vi "Update VS channels - incoming - (object info).vi"(9 "reflectAttributeValues in":T1, 10 "hla map helpers in":T7, 11 "values in":dbl[](array[numeric])) -> (1 "reflectAttributeValues out":T1, 2 "hla map helpers out":T7, 3 "values out":dbl[](array[numeric]))   [LabVIEW 2019, in "HLA Custom Device Engine.lvlib"]
uses:
  HLA Custom Device Engine.lvlib
  _typedefs/RThlaMapHelpers.ctl
  _typedefs/map_in_interaction.ctl
  _typedefs/map_interaction_value.ctl
  _typedefs/map_attr_param_data.ctl
  _typedefs/map_object.ctl
  _typedefs/map_object_key.ctl
  _typedefs/map_object_value.ctl
  _typedefs/map_object_instance.ctl
  _typedefs/map_object_instance_value.ctl
  _typedefs/map_object_vs_instance.ctl
  _typedefs/map_out_vs_ch_instanceId.ctl
  _typedefs/map_out_vs_ch_objects.ctl
  _typedefs/map_out_vs_ch_objects_value.ctl
  _typedefs/map_out_vs_ch_interactIonClass.ctl
  _typedefs/reflectAttributeValues_type.ctl
  _typedefs/object_info_received_type.ctl
  <vilib>/addons/hla/TransportationType.ctl
  <vilib>/addons/hla/OrderType.ctl
  Shared/vs_obj_id_state.ctl
  _typedefs/dataElement_type.ctl
  _Debug/VsDebugLibrary.lvlib
  <vilib>/addons/hla/openrti_rti1516eLv.lvlib
  Shared/HLA Custom Device Shared.lvlib
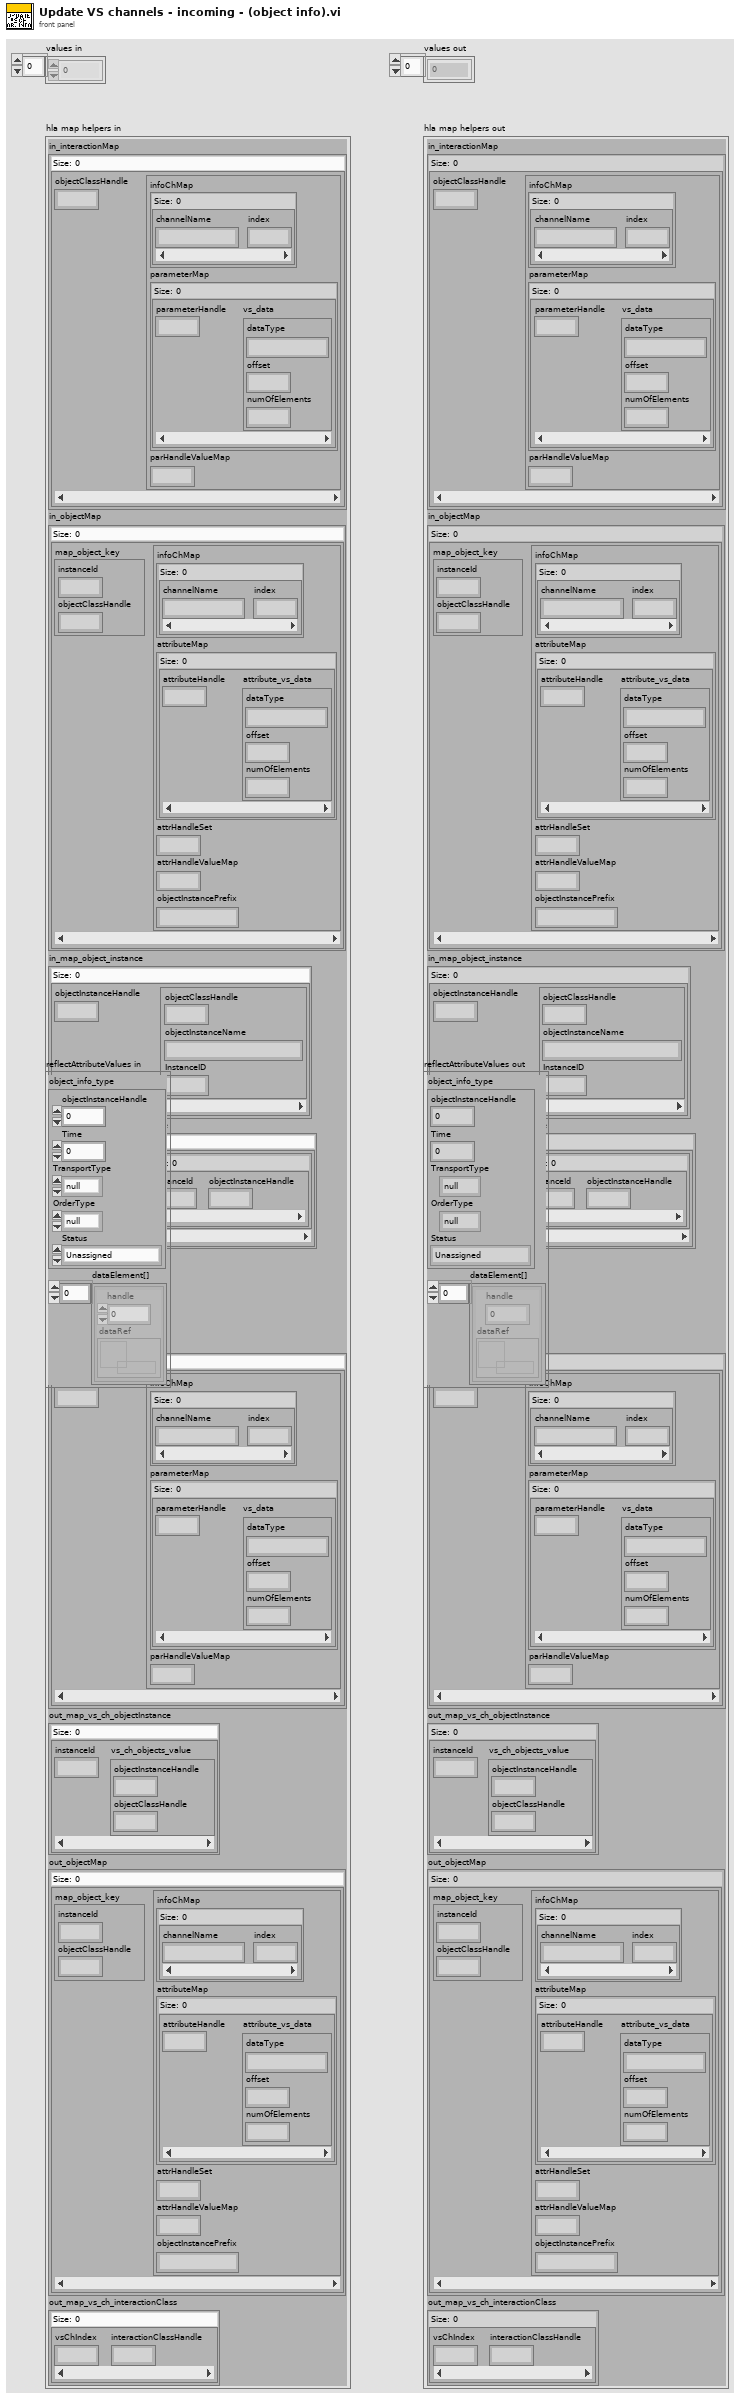
[diagram p1: front panel]
types:
  T1 = typedef "HLA Custom Device Engine.lvlib/reflectAttributeValues_type.ctl" = cluster{"object_info_type":T2, "dataElement[]":T6[]}
  T2 = typedef "HLA Custom Device Engine.lvlib/object_info_received_type.ctl" = cluster{"objectInstanceHandle":u64, "Time":dbl, "TransportType":T3, "OrderType":T4, "Status":T5}
  T3 = typedef "openrti_rti1516eLv.lvlib/TransportationType.ctl" = enum32{"null", "RELIABLE", "BEST_EFFORT"}
  T4 = typedef "openrti_rti1516eLv.lvlib/OrderType.ctl" = enum32{"null", "RECEIVE", "TIMESTAMP"}
  T5 = typedef "HLA Custom Device Shared.lvlib/vs_obj_id_state.ctl" = enum16{"Unassigned", "Assigned", "Removed"}
  T6 = typedef "HLA Custom Device Engine.lvlib/dataElement_type.ctl" = cluster{"handle":u64, "dataRef":refnum<data-value>}
  T7 = typedef "HLA Custom Device Engine.lvlib/RThlaMapHelpers.ctl" = cluster{"in_interactionMap":T8, "in_objectMap":T11, "in_map_object_instance":T14, "in_map_vs_incoming_instance":T16, "out_map_vs_ch_instanceId":T17, "out_interactionMap":T8, "out_map_vs_ch_objectInstance":T18, "out_objectMap":T11, "out_map_vs_ch_interactionClass":T20}
  T8 = typedef "HLA Custom Device Engine.lvlib/map_in_interaction.ctl" = map{u64, T9}
  T9 = typedef "HLA Custom Device Engine.lvlib/map_interaction_value.ctl" = cluster{"infoChMap":map{string, i32}, "parameterMap":map{u64, T10}, "parHandleValueMap":u64}
  T10 = typedef "HLA Custom Device Engine.lvlib/map_attr_param_data.ctl" = cluster{"dataType":string, "offset":i32, "numOfElements":i32}
  T11 = typedef "HLA Custom Device Engine.lvlib/map_object.ctl" = map{T12, T13}
  T12 = typedef "HLA Custom Device Engine.lvlib/map_object_key.ctl" = cluster{"instanceId":i32, "objectClassHandle":u64}
  T13 = typedef "HLA Custom Device Engine.lvlib/map_object_value.ctl" = cluster{"infoChMap":map{string, i32}, "attributeMap":map{u64, T10}, "attrHandleSet":u64, "attrHandleValueMap":u64, "objectInstancePrefix":string}
  T14 = typedef "HLA Custom Device Engine.lvlib/map_object_instance.ctl" = map{u64, T15}
  T15 = typedef "HLA Custom Device Engine.lvlib/map_object_instance_value.ctl" = cluster{"objectClassHandle":u64, "objectInstanceName":string, "InstanceID":i32}
  T16 = typedef "HLA Custom Device Engine.lvlib/map_object_vs_instance.ctl" = map{u64, map{i32, u64}}
  T17 = typedef "HLA Custom Device Engine.lvlib/map_out_vs_ch_instanceId.ctl" = map{i32, i32}
  T18 = typedef "HLA Custom Device Engine.lvlib/map_out_vs_ch_objects.ctl" = map{i32, T19}
  T19 = typedef "HLA Custom Device Engine.lvlib/map_out_vs_ch_objects_value.ctl" = cluster{"objectInstanceHandle":u64, "objectClassHandle":u64}
  T20 = typedef "HLA Custom Device Engine.lvlib/map_out_vs_ch_interactIonClass.ctl" = map{i32, u64}
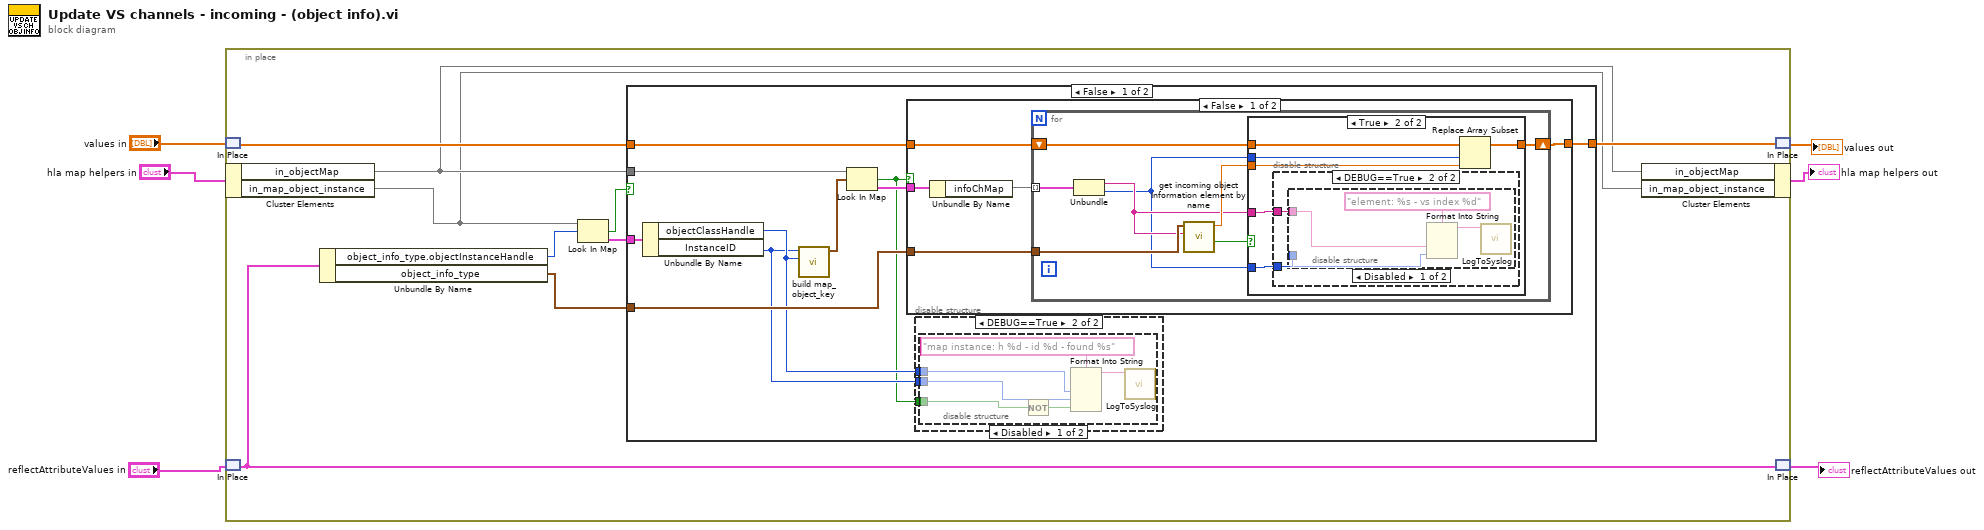
[diagram p0: block diagram]
diagram:
  n1 = in-place {
    n2 = in-place-match #1("values in") -> (w15:dbl[])
    n3 = in-place-cluster #2("hla map helpers in") -> ("in_objectMap"=w13:T11, "in_map_object_instance"=w10:T14)
    n4 = in-place-match #3("reflectAttributeValues in") -> (w12:T1)
    n5 = Unbundle By Name(w12) -> ("object_info_type.objectInstanceHandle"=w11:u64, "object_info_type"=w7:T2)
    n6 = Look In Map(map=w10, key=w11) -> (key not found?=w9:bool, value=w8:T15)  [unwired: 1 in]
    n7 = case shown="False" w9 {
      tunnel: w15 -> [w24 w62]
      tunnel: [w23 w62] -> w14
      tunnel: w13 -> [w22 _]
      tunnel: w7 -> [w21 _]
      tunnel: w8 -> [w20 _]
      frame False {
        n8 = Unbundle By Name(w20) -> ("objectClassHandle"=w18:u64, "InstanceID"=w17:i32)
        n9 = call "build map_object_key.vi"("objectClassHandle"=w18, "instanceId"=w17) -> ("object_map_key"=w19:T12)  [unwired: 9 in]
        n10 = Look In Map(map=w22, key=w19) -> (key not found?=w16:bool, value=w25:T13)  [unwired: 1 in]
        n11 = case shown="False" w16 {
          tunnel: [w38 w61] -> w23
          tunnel: w25 -> [w36 _]
          tunnel: w24 -> [w37 w61]
          tunnel: w21 -> [w35 _]
          frame False {
            n12 = Unbundle By Name(w36) -> ("infoChMap"=w39:map{string, i32})
            n13 = for {
              tunnel: w39 -> [w43] mode=indexing
              shift-right: [w46] -> w38
              shift-left: w37 -> [w47]
              tunnel: w35 -> [w42]
              n14 = Unbundle(w43) -> ("channelName"=w41:string, "index"=w40:i32)
              n15 = call "get incoming object Information element by name.vi"("name"=w41, "interaction_attribute_type"=w42) -> ("found"=w44:bool, "element out"=w45:dbl)  [unwired: 8 in]
              n16 = case shown="True" w44 {
                tunnel: w47 -> [w48 w54]
                tunnel: [w48 w53] -> w46
                tunnel: w45 -> [_ w52]
                tunnel: w40 -> [_ w51]
                tunnel: w41 -> [_ w50]
                tunnel: w40 -> [_ w49]
                frame False {
                }
                frame True {
                  n17 = disable-structure shown="DEBUG==True" {
                    disable-tunnel: w50 -> [_ w56]
                    disable-tunnel: w49 -> [_ w55]
                    frame condition #0 {
                    }
                    frame condition #1 (active) {
                      n18 = disable-structure shown="Disabled" {
                        disable-tunnel: w56 -> [w58 _]
                        disable-tunnel: w55 -> [w57 _]
                        frame Disabled {
                          n19 = Format Into String(format string="element: %s - vs index %d" ("message"), w58, w57) -> (resulting string=w59:string)  [unwired: 2 in, 1 out]
                          n20 = call "LogToSyslog.vi"("message"=w59) -> ()  [unwired: 9 in, 2 out]
                        }
                        frame Enabled {
                        }
                      }
                    }
                  }
                  n21 = Replace Array Subset(array=w54, new element=w52, index=w51) -> (w53:dbl[])
                }
              }
            }
          }
          frame True {
          }
        }
        n22 = disable-structure shown="DEBUG==True" {
          disable-tunnel: w17 -> [_ w26]
          disable-tunnel: w18 -> [_ w27]
          disable-tunnel: w16 -> [_ w28]
          frame condition #0 {
          }
          frame condition #1 (active) {
            n23 = disable-structure shown="Disabled" {
              disable-tunnel: w28 -> [w32 _]
              disable-tunnel: w27 -> [w31 _]
              disable-tunnel: w26 -> [w30 _]
              frame Disabled {
                n24 = Not(x=w32) -> (.not. x?=w29:bool)
                n25 = Format Into String(format string="map instance: h %d - id %d - found %s" ("message"), w31, w30, w29) -> (resulting string=w33:string)  [unwired: 2 in, 1 out]
                n26 = call "LogToSyslog.vi"("message"=w33) -> ()  [unwired: 9 in, 2 out]
              }
              frame Enabled {
              }
            }
          }
        }
      }
      frame True {
      }
    }
    n27 = in-place-cluster #2("in_objectMap"=w13, "in_map_object_instance"=w10) -> (→"hla map helpers out":T7)
    n28 = in-place-match #1(w14) -> (→"values out":dbl[])
    n29 = in-place-match #3(w12) -> (→"reflectAttributeValues out":T1)
  }
